vi "GenesysPS.SetOnOff.vi"(0 "i ref in":refnum<vi>, 2 "on (FALSE)":bool, 5 "error in (no error)":errorcluster) -> (14 "i ref out":refnum<vi>, 19 "error out":errorcluster)   [LabVIEW 2014, in "GenesysPS.lvlib"]
doc: "Switches the PS on and off (command send via RS485).\n\nLicense Agreement for this software:\n\nCopyright (C)\nGesellschaft für Schwerionenforschung, GSI\nPlanckstr. 1\n64291 Darmstadt\nGermany\n\nContact: D.Beck@gsi.de \n\nThis program is free software; you can redistribute it and/or modify it under the terms of the GNU General Public License as published by the Free Software Foundation; either version 2 of the license, or (at your option) any later version.\n\nThis program is distributed in the hope that it will be useful, but WITHOUT ANY WARRANTY; without even the implied warranty of MERCHANTABILITY or FITNESS FOR A PARTICULAR PURPOSE. See the GNU General License for more details (http://www.gnu.org).\n\nGesellschaft für Schwerionenforschung, GSI\nPlanckstr. 1, 64291 Darmstadt, Germany\nFor all questions and ideas contact: M.Richter@gsi.de, H.Brand@gsi.de or D.Beck@gsi.de.\nLast update: 17-JUN-2004"
uses:
  GenesysPS.lvlib
  CSinstr.lib/GENser/GENserDriver.lvlib
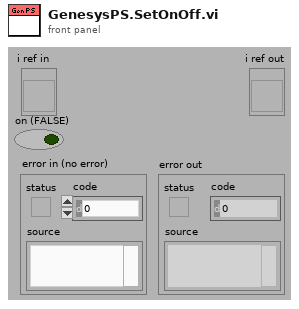
[diagram p1: front panel]
types:
  T1 = typedef "GenesysPS.lvlib/GenesysPS.i attribute.ctl" = cluster{"VISA name/ Heizinger":refnum<visa-resource-name>, "GEN Addr":i32, "WithTempInt?":bool, "TempLimit":dbl, "TemperatureID":i32, "Temp queue":refnum<queue>}
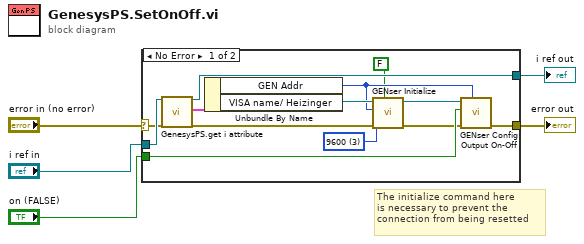
[diagram p0: block diagram]
diagram:
  # "The initialize command here\nis necessary to prevent the\nconnection from being resetted"
  n1 = case shown="No Error" "error in (no error)" {
    selector: "error in (no error)" -> [w17 w20]
    tunnel: [w15 w20] -> w5
    tunnel: [w14 w19] -> w3
    tunnel: "i ref in" -> [w18 w19]
    tunnel: "on (FALSE)" -> [w13 _]
    frame No Error {
      w7 = u16 3 items=["1200", "2400", "4800", "9600", "19200"] ("BAUD")
      n2 = call "GenesysPS.get i attribute.vi"("i ref in"=w18, "error in (no error)"=w17) -> ("i ref out"=w14:refnum<vi>, "i attribute"=w16:T1, "error out"=w9:errorcluster)  [unwired: 15 in]
      n3 = Unbundle By Name(w16) -> ("GEN Addr"=w8:i32, "VISA name/ Heizinger"=w10:refnum<visa-resource-name>)
      n4 = call "GENser Initialize.vi"("Reset (T)"=FALSE, "error in (no error)"=w9, "BAUD"=w7, "GEN Addr"=w8, "VISA name"=w10) -> ("error out"=w12:errorcluster, "VISA out"=w11:refnum<visa-resource-name>)  [unwired: 5 in]
      n5 = call "GENser Config Output On-Off.vi"("GEN Addr"=w8, "error"=w12, "Output ON"=w13, "VISA"=w11) -> ("error out"=w15:errorcluster)  [unwired: 6 in, 1 out]
    }
    frame Error {
    }
  }
  "i ref out" <- w3
  "error out" <- w5
